vi "change tag data type.vi"(7 "data type":T1, 8 "error in":errorcluster, 10 "tag name":string, 11 "shared memory module configuration in":refnum<class "Shared Memory Configuration.lvclass">) -> (0 "error out":errorcluster, 2 "changed channels":refnum<class "TBM channel.lvclass">[](array[class]), 3 "shared memory module configuration out":refnum<class "Shared Memory Configuration.lvclass">)   [LabVIEW 2013, in "Shared Memory Configuration.lvclass"]
doc: "Copyright 2016 National Instruments Corporation\n\nLicensed under the Apache License, Version 2.0 (the \"License\"); you may not use this file except in compliance with the License. You may obtain a copy of the License at http://www.apache.org/licenses/LICENSE-2.0\nUnless required by applicable law or agreed to in writing, software distributed under the License is distributed on an \"AS IS\" BASIS, WITHOUT WARRANTIES OR CONDITIONS OF ANY KIND, either express or implied. See the License for the specific language governing permissions and limitations under the License."
uses:
  Shared Memory Configuration.lvclass
  <vilib>/NI/Tag Bus/tag/Data Type.ctl
  <vilib>/NI/Tag Bus Module Framework/channel/TBM channel.lvclass
  <vilib>/NI/Tag Bus/tag/tag descriptor.lvclass/tag descriptor.ctl
  Shared Memory Configuration.lvclass/Shared Memory Configuration.ctl
  <vilib>/NI/Tag Bus/tag/tag descriptor.lvclass
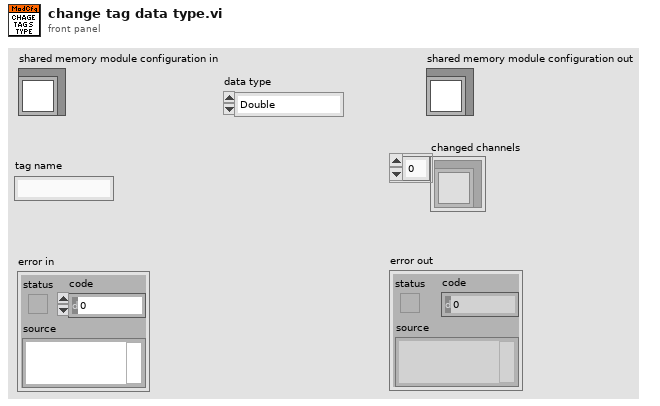
[diagram p1: front panel]
types:
  T1 = typedef "tag bus.lvlib/tag descriptor.lvclass/Data Type.ctl" = enum16{"Double", "Single", "I64", "I32", "I16", "I8", "U64", "U32", "U16", "U8", "Boolean", "String", "Array of Double", "Array of Single", "Array of I64", "Array of I32", "Array of I16", "Array of I8", "Array of U64", "Array of U32", "Array of U16", "Array of U8", "Array of Boolean", "Array of String"}
  T2 = typedef "Shared Memory Configuration.lvclass/line configuration.ctl" = cluster{"name":string, "data type":T1, "channel":refnum<class "TBM channel.lvclass">}
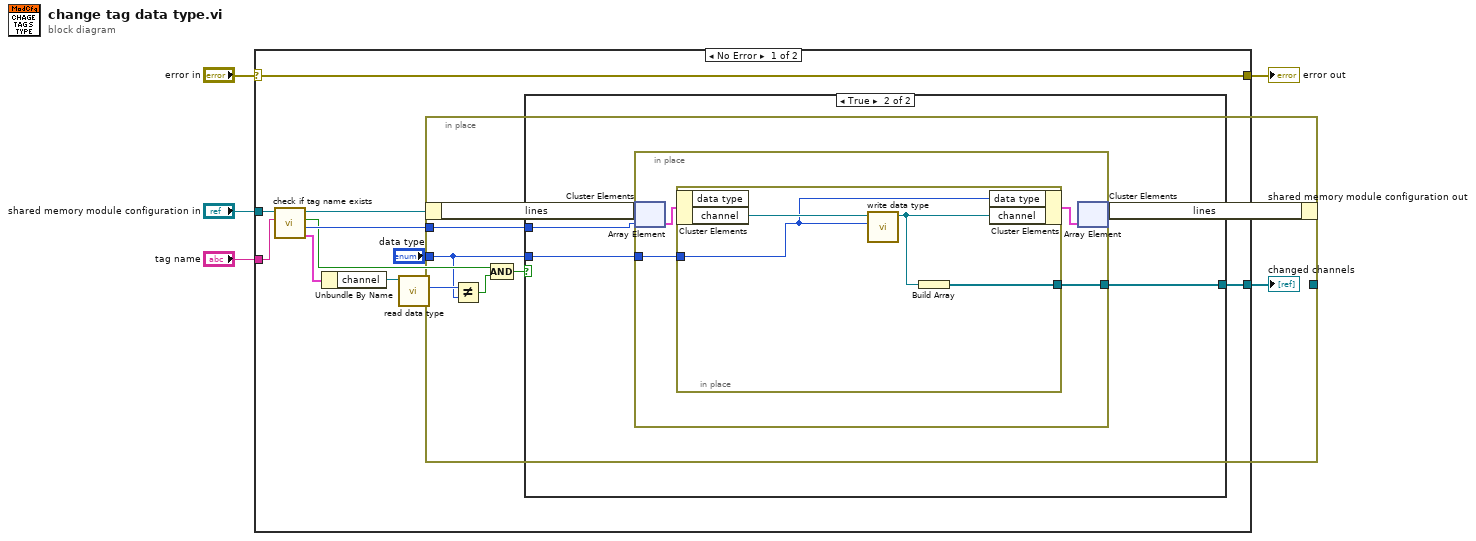
[diagram p0: block diagram]
diagram:
  n1 = case shown="No Error" "error in" {
    selector: "error in" -> [w7 w41]
    tunnel: "shared memory module configuration in" -> [w20 w40]
    tunnel: "tag name" -> [w19 _]
    tunnel: [w10 _] -> w5
    tunnel: [w9 w40] -> w4
    tunnel: [w7 w41] -> w2
    frame No Error {
      n2 = call "check if tag name exists.vi"("name to locate"=w19, "shared memory module configuration in"=w20) -> ("tag config"=w16:T2, "index"=w17:i32, "found?"=w13:bool, "shared memory module configuration out"=w18:refnum<class "Shared Memory Configuration.lvclass">)  [unwired: 6 in]
      n3 = Unbundle By Name(w16) -> ("channel"=w15:refnum<class "TBM channel.lvclass">)
      n4 = call <vilib>:"read data type.vi"("system tag in"=w15) -> ("data type"=w14:T1)  [unwired: 8 in, 2 out]
      n5 = Not Equal?(x=w14, y="data type") -> (x != y?=w12:bool)
      n6 = Compound Arithmetic op=AND(w13, w12) -> (w11:bool)
      n7 = case shown="True" w11 {
        tunnel: w18 -> [w21 w26]
        tunnel: [w21 w25] -> w9
        tunnel: w17 -> [_ w24]
        tunnel: [_ w23] -> w10
        tunnel: "data type" -> [_ w22]
        frame False {
        }
        frame True {
          n8 = in-place {
            in-place-border: w24 -> [w29]
            in-place-border: [w28] -> w23
            in-place-border: w22 -> [w27]
            n9 = in-place-cluster #1(w26) -> ("lines"=w31:T2[])
            n10 = in-place {
              in-place-border: [w33] -> w28
              in-place-border: w27 -> [w32]
              n11 = in-place-array #2(w31, w29) -> (w35:T2)
              n12 = in-place {
                in-place-border: [w39] -> w33
                in-place-border: w32 -> [w36]
                n13 = in-place-cluster #3(w35) -> ("channel"=w38:refnum<class "TBM channel.lvclass">)  [unwired: 1 out]
                n14 = call <vilib>:"write data type.vi"("data type"=w36, "system tag in"=w38) -> ("system tag out"=w37:refnum<class "TBM channel.lvclass">)  [unwired: 8 in, 1 out]
                n15 = Build Array(w37) -> (w39:refnum<class "TBM channel.lvclass">[])
                n16 = in-place-cluster #3("data type"=w36, "channel"=w37) -> (w34:T2)
              }
              n17 = in-place-array #2(w34) -> (w30:T2[])  [unwired: 1 out]
            }
            n18 = in-place-cluster #1("lines"=w30) -> (w25:refnum<class "Shared Memory Configuration.lvclass">)
          }
        }
      }
    }
    frame Error {
    }
  }
  "error out" <- w2
  "shared memory module configuration out" <- w4
  "changed channels" <- w5
